vi "plot-nameSD.vi"(0 "plot names in":string[](array[string]), 1 "To":dbl, 2 "exp selected":i32, 3 "Item Names":string[](array[string]), 4 "from":dbl) -> (5 "plot names out":string[](array[string]))   [LabVIEW 2015]
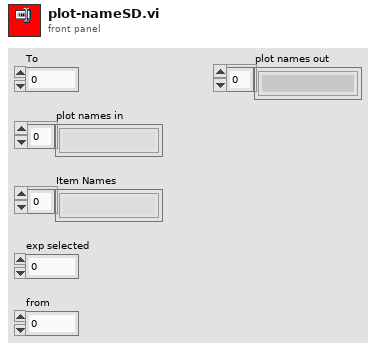
[diagram p1: front panel]
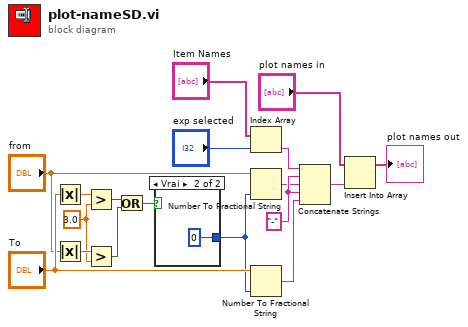
[diagram p0: block diagram]
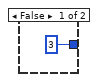
[diagram p2: hidden frame]
diagram:
  w5 = 3.0 ("y")
  w14 = "-" ("string")
  n1 = Absolute Value(x="To") -> (abs(x)=w9:dbl)
  n2 = Absolute Value(x="from") -> (abs(x)=w6:dbl)
  n3 = Greater?(x=w9, y=w5) -> (0:w4:bool)
  n4 = Greater?(x=w6, y=w5) -> (0:w3:bool)
  n5 = Or(x=w4, y=w3) -> (x .or. y?=w2:bool)
  n6 = case shown="Vrai" w2 {
    tunnel: [i16 3 ("precision (6)") i16 0 ("precision (6)")] -> w1
    frame False {
    }
    frame True {
    }
  }
  n7 = Index Array(array="Item Names", index="exp selected") -> (element=w17:string)
  n8 = Number To Fractional String(number="from", precision (6)=w1) -> (F-format string=w10:string)  [unwired: 2 in]
  n9 = Number To Fractional String(number="To", precision (6)=w1) -> (F-format string=w11:string)  [unwired: 2 in]
  n10 = Concatenate Strings(w17, w14, w10, w14, w11) -> (w18:string)
  n11 = Insert Into Array(array="plot names in", new element=w18) -> (→"plot names out":string[])  [unwired: 1 in]
